vi "Test MQTT-6.0.0-3.vi"(8 "error in (no error)":errorcluster, 11 "Connection Config":refnum<class "Connection.lvclass">) -> (0 "error out":errorcluster, 3 "Connection Config dup":refnum<class "Connection.lvclass">)   [LabVIEW 2013]
uses:
  <vilib>/LabVIEW Open Source Project/MQTT Connection/MQTT_Connection/Connection/Connection.lvclass
  <vilib>/LabVIEW Open Source Project/MQTT Websockets Connection/MQTT_Websockets/Connection/WebsocketsConnection.lvclass
  <vilib>/addons/_JKI Toolkits/Caraya/classes/Test/Test.lvclass
  <vilib>/addons/_JKI Toolkits/Caraya/classes/Assert/Assert.lvclass
panel:
  out "Return Headers":variant
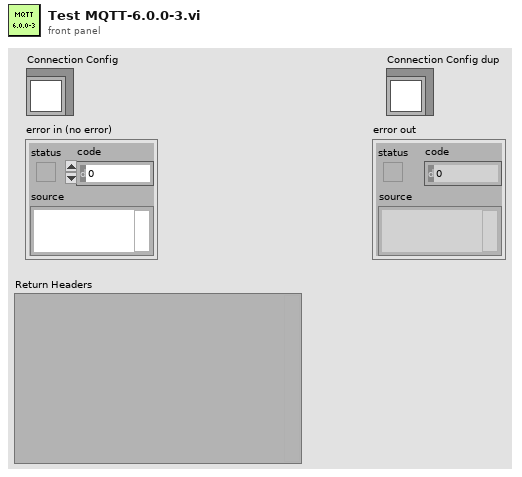
[diagram p1: front panel]
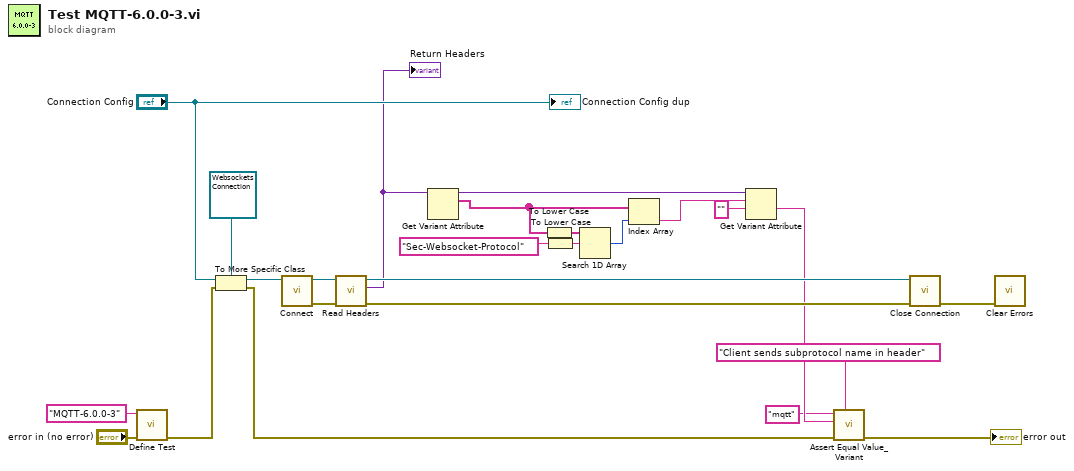
[diagram p0: block diagram]
diagram:
  n1 = call <vilib>:"Define Test.vi"("error in (no error)"="error in (no error)", "Label (VI Title)"="MQTT-6.0.0-3") -> ("error out"=w10:errorcluster)  [unwired: 9 in]
  n2 = To More Specific Class(target class=refnum<class "WebsocketsConnection.lvclass"> refnum ("WebsocketsConnection in"), reference="Connection Config", error in=w10) -> (specific class reference=w11:refnum<class "WebsocketsConnection.lvclass">, error out=w9:errorcluster)
  n3 = call <vilib>:"Connect.vi"("Connection in"=w11) -> ("error out"=w17:errorcluster, "Connection out"=w18:refnum<class "WebsocketsConnection.lvclass">)  [unwired: 9 in]
  n4 = call <vilib>:"Read Headers.vi"("error in (no error)"=w17, "WebsocketsConnection in"=w18) -> ("error out"=w15:errorcluster, "Return Headers"=w8:variant, "WebsocketsConnection out"=w16:refnum<class "WebsocketsConnection.lvclass">)  [unwired: 7 in]
  "Return Headers" <- w8
  n5 = Get Variant Attribute(Variant=w8) -> (duplicate Variant=w7:variant, names=w1:string[])  [unwired: 3 in, 2 out]
  n6 = To Lower Case(string=w1) -> (all lower case string=w6:string[])
  n7 = To Lower Case(string="Sec-Websocket-Protocol" ("name")) -> (all lower case string=w5:string)
  n8 = Search 1D Array(1D array=w6, element=w5) -> (index of element=w3:i32)  [unwired: 1 in]
  n9 = Index Array(array=w1, index=w3) -> (element=w2:string)
  n10 = Get Variant Attribute(Variant=w7, name=w2, default value (empty Variant)="") -> (value=w13:string)  [unwired: 1 in, 3 out]
  n11 = call <vilib>:"Assert Equal Value_Variant.vi"("Label"="Client sends subprotocol name in header", "error in (no error)"=w9, "Y"=w13, "X"="mqtt") -> ("error out"=→"error out":errorcluster)  [unwired: 7 in]
  n12 = call <vilib>:"Close Connection.vi"("error in (no error)"=w15, "Connection in"=w16) -> ("error out"=w19:errorcluster)  [unwired: 8 in, 1 out]
  n13 = call <vilib>:"Clear Errors.vi"("error in (no error)"=w19) -> ()  [unwired: 6 in, 1 out]
  "Connection Config dup" <- "Connection Config"
